vi "HandleCollector.vi"(9 "Lower Collector?":bool, 10 "Raise Collector?":bool) -> (1 "CollectorEnum Input":T1)   [LabVIEW 2013]
doc: "Takes in two booleans of whether to raise or lower the collector, and the outpus the enum \"Raise\", \"Lower\", or \"Stop\""
uses:
  CollectorEnum.ctl
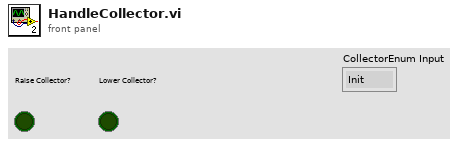
[diagram p1: front panel]
types:
  T1 = typedef "CollectorEnum.ctl" = enum16{"Init", "Raise", "Lower", "Stop", "GetStatus"}
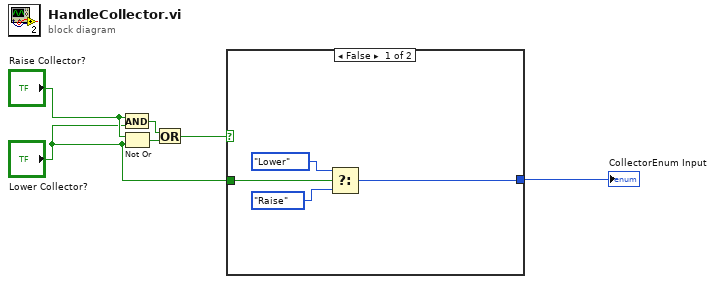
[diagram p0: block diagram]
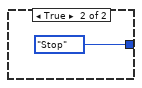
[diagram p2: hidden frame]
diagram:
  n1 = And(x="Raise Collector?", y="Lower Collector?") -> (x .and. y?=w3:bool)
  n2 = Not Or(1:"Lower Collector?", 2:"Raise Collector?") -> (0:w2:bool)
  n3 = Or(x=w3, y=w2) -> (x .or. y?=w4:bool)
  n4 = case shown="False" w4 {
    tunnel: [w7 CollectorEnum."Stop" ("Enum")] -> w6
    tunnel: "Lower Collector?" -> [w10 _]
    frame False {
      n5 = Select(t=CollectorEnum."Lower" ("Enum"), s=w10, f=CollectorEnum."Raise" ("Enum")) -> (s? t:f=w7:T1)
    }
    frame True {
    }
  }
  "CollectorEnum Input" <- w6
